vi "Check Status (No Objects).vi"(8 "error in (no error)":errorcluster, 11 "Cluster In":T1) -> (0 "error out":errorcluster, 1 "Status":string, 2 "Ready?":bool, 3 "Cluster Out":T1)   [LabVIEW 2009]
doc: "(Dynamic) Check if the instrument is powered on and update its member fields with the instrument's current status. Optionally return a text status message."
uses:
  Global/GPIB Numbers.vi
  BEOC LPC/BEOC LPC.lvlib
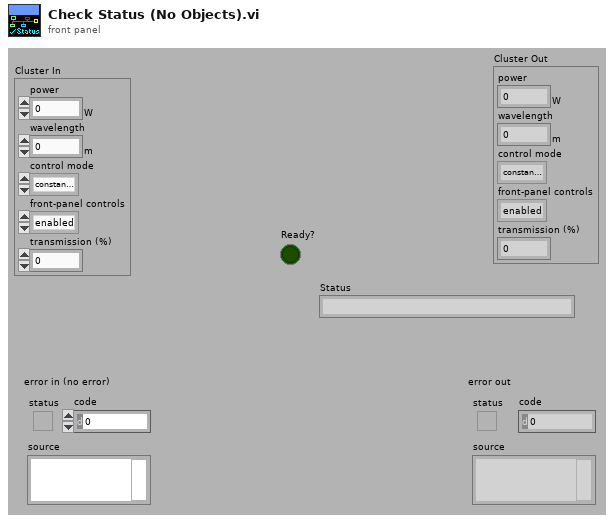
[diagram p1: front panel]
types:
  T1 = cluster{"power":dbl[unit], "wavelength":dbl[unit], "control mode":enum16{"constant power", "constant transmission"}, "front-panel controls":enum16{"enabled", "disabled"}, "transmission (%)":dbl}
  T2 = typedef "GPIB Type Def.ctl" = cluster{"Name":string, "bus":dbl, "GPIB":dbl, "GPIB as string":string, "byte":i32, "VISA Resource Name":refnum<visa-resource-name>}
  T3 = enum16{"constant power", "constant transmission"}
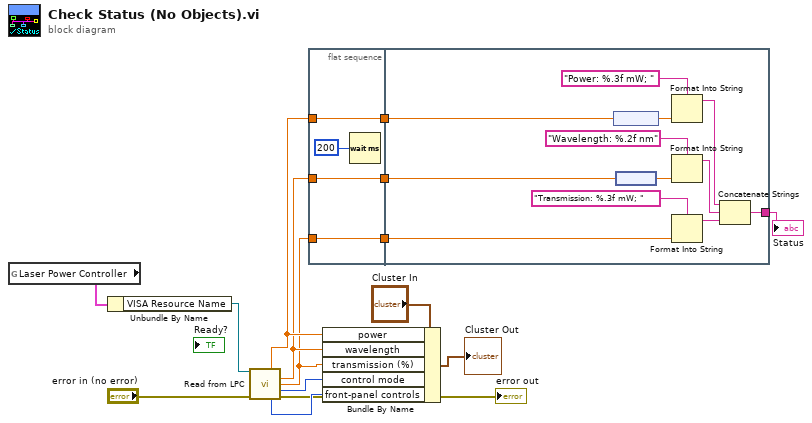
[diagram p0: block diagram]
diagram:
  n1 = global read "GPIB Numbers.vi" "Laser Power Controller"() -> (w3:T2)
  n2 = Unbundle By Name(w3) -> ("VISA Resource Name"=w2:refnum<visa-resource-name>)
  n3 = call "Read from LPC.vi"("VISA resource name"=w2, "error in (no error)"="error in (no error)") -> ("power"=w13:dbl[unit], "wavelength"=w12:dbl[unit], "Transmission"=w10:dbl, "control mode"=w15:T3, "front-panel controls"=w14:enum16{"enabled", "disabled"}, "error out"=→"error out":errorcluster)  [unwired: 7 in, 1 out]
  n4 = flat-sequence {
    tunnel: w10 -> [w17]
    tunnel: w12 -> [w18]
    tunnel: w13 -> [w19]
    tunnel: [w19] -> w9
    tunnel: [w18] -> w8
    tunnel: [w17] -> w7
    tunnel: [w25] -> w11
    tunnel: w9 -> [w31]
    tunnel: w8 -> [w29]
    tunnel: w7 -> [w20]
    frame #0 {
      n5 = Wait (ms)(milliseconds to wait=u32 200) -> ()  [unwired: 1 out]
    }
    frame #1 {
      n6 = node(w31) -> (w24:dbl)
      n7 = node(w29) -> (w23:dbl)
      n8 = Format Into String(format string="Power: %.3f mW; ", w24) -> (resulting string=w26:string)  [unwired: 2 in, 1 out]
      n9 = Format Into String(format string="Wavelength: %.2f nm", w23) -> (resulting string=w27:string)  [unwired: 2 in, 1 out]
      n10 = Format Into String(format string="Transmission: %.3f mW; ", w20) -> (resulting string=w21:string)  [unwired: 2 in, 1 out]
      n11 = Concatenate Strings(w26, w27, w21) -> (w25:string)
    }
  }
  n12 = Bundle By Name(cluster="Cluster In", "power"=w13, "wavelength"=w12, "transmission (%)"=w10, "control mode"=w15, "front-panel controls"=w14) -> (→"Cluster Out":T1)
  "Status" <- w11
